vi "Initialize.vi"(6 "Reset (True)":bool=TRUE, 7 "Serial Configuration":T1={"Baud Rate"=9600, "Parity"=0, "Data Bits"=7, "Stop Bits"=10, "Flow Control"=0} {"Flow Control" items=["None", "XON/XOFF", "RTS/CTS", "XON/XOFF & RTS/CTS", "DTR/DSR", "XON/XOFF & DTR/DSR"]; "Stop Bits" items=["1.0"=10, "1.5"=15, "2.0"=20]; "Data Bits" items=["7"=7, "8"=8]; "Parity" items=["None", "Odd", "Even", "Mark", "Space"]; "Baud Rate" items=["300"=300, "600"=600, "1200"=1200, "2400"=2400, "4800"=4800, "9600"=9600, "19200"=19200]}, 8 "error in (no error)":errorcluster, 9 "Error Query (False)":bool, 10 "ID Query (True)":bool=TRUE, 11 "VISA resource name":refnum<visa-resource-name>) -> (0 "error out":errorcluster, 3 "VISA resource name out":refnum<visa-resource-name>)   [LabVIEW 2018, in "Keithley 2600 Series.lvlib"]
doc: "Establishes communication with the instrument and optionally performs an instrument identification query and/or an instrument reset. It also places the instrument in a default state needed for other instrument driver operations. Therefore, call this VI before calling other instrument driver VIs for this instrument. Generally, you need to call the Initialize VI only once at the beginning of an application."
uses:
  Keithley 2600 Series.lvlib
  GlobalVariables.vi
panel:
  # "(c) 2008 Keithley Instruments, Inc.  ALL RIGHTS RESERVED."
  # "Automatic"
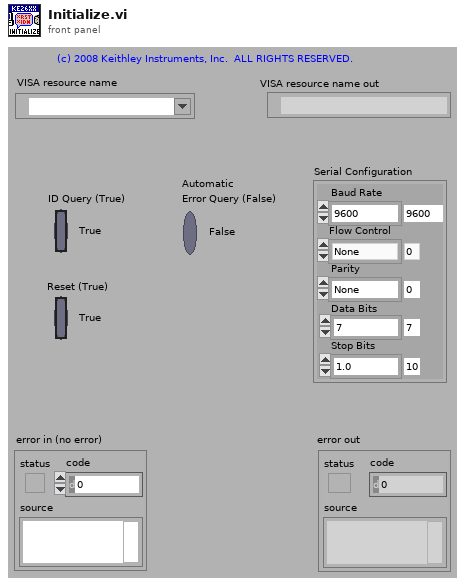
[diagram p1: front panel]
types:
  T1 = cluster{"Baud Rate":u32, "Parity":u16, "Data Bits":u16, "Stop Bits":u16, "Flow Control":u16}
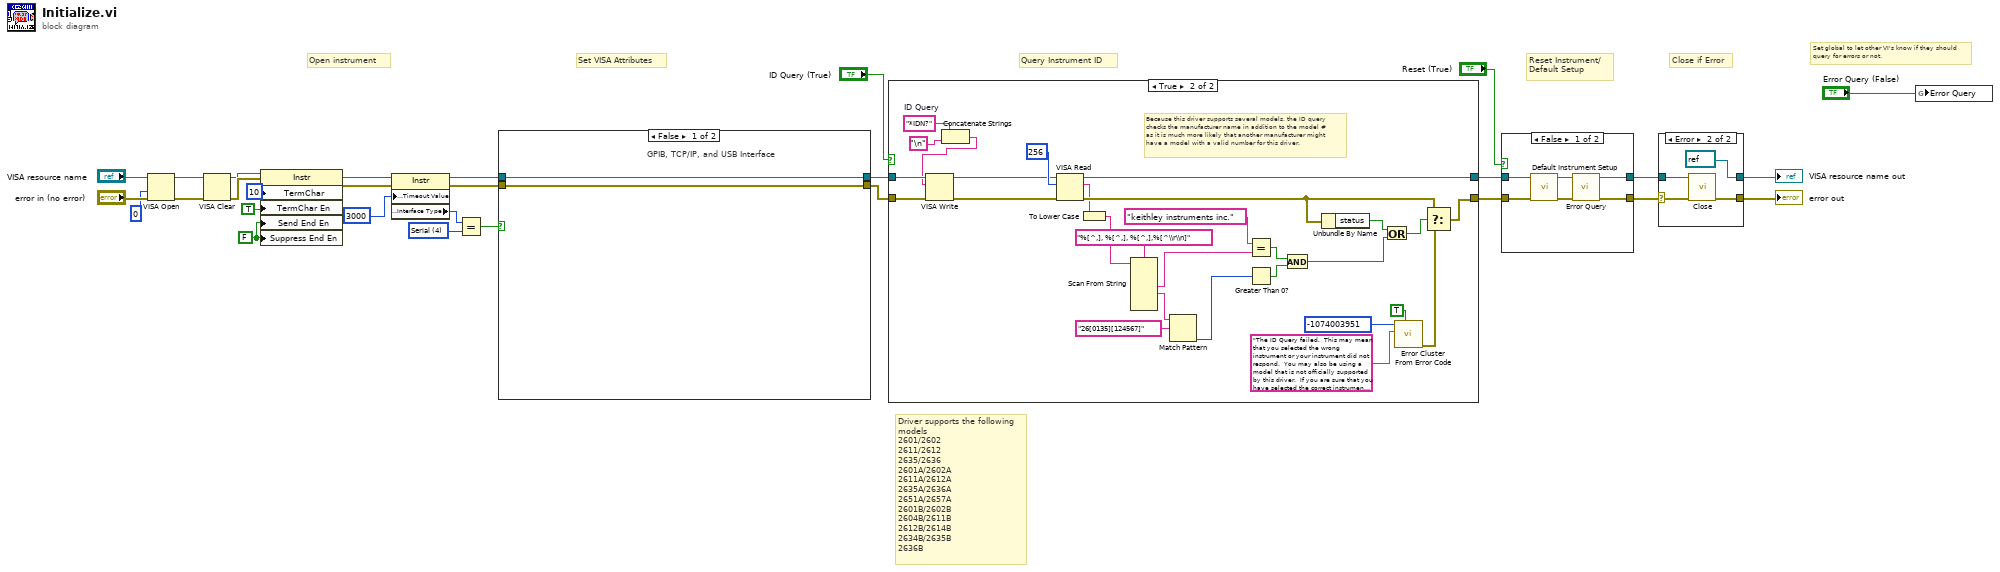
[diagram p0: block diagram]
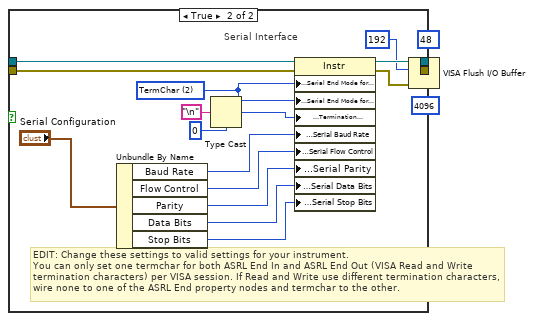
[diagram p2: hidden frame]
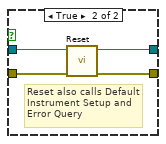
[diagram p4: hidden frame]
diagram:
  w1 = FALSE ("Message Based Settings:Suppress End Enable")
  w16 = u16 4 items=["GPIB"=1, "VXI"=2, "GPIB-VXI"=3, "Serial"=4, "PXI"=5, "TCPIP"=6, "USB"=7] ("Interface Information:Interface Type")
  # "Driver supports the following models\n2601/2602\n2611/2612\n2635/2636\n2601A/2602A\n2611A/2612A\n2635A/2636A\n2651A/2657A\n2601B/2602B\n2604B/2611B\n2612B/2614B\n2634B/2635B\n2636B"
  # "Set global to let other VI's know if they should\nquery for errors or not."
  # "Set VISA Attributes"
  # "Close if Error"
  # "Query Instrument ID"
  # "Reset Instrument/\nDefault Setup"
  # "Open instrument"
  n1 = VISA Open(access mode=u32 0, error in (no error)="error in (no error)", VISA resource name="VISA resource name") -> (VISA resource name=w14:refnum<visa-resource-name>, error out=w13:errorcluster)  [unwired: 2 out]
  n2 = VISA Clear(VISA resource name=w14, error in (no error)=w13) -> (VISA resource name out=w4:refnum<visa-resource-name>, error out=w5:errorcluster)
  n3 = property class="Instr"(reference=w4, error in=w5, "TermChar"=u8 10 ("Message Based Settings:Termination Character"), "TermChar En"=TRUE ("Message Based Settings:Termination Character Enable"), "Send End En"=w1, "Suppress End En"=w1) -> (reference out=w3:refnum<visa-resource-name>, error out=w2:errorcluster)
  n4 = property class="Instr"(reference=w3, error in=w2, "General Settings:Timeout Value"=u32 3000) -> (reference out=w19:refnum<visa-resource-name>, error out=w18:errorcluster, "Interface Information:Interface Type"=w23:u16)
  n5 = Equal?(x=w23, y=w16) -> (x = y?=w17:bool)
  n6 = case shown="False" w17 {
    tunnel: [w30 w49] -> w21
    tunnel: [w31 w46] -> w20
    tunnel: w19 -> [w30 w51]
    tunnel: w18 -> [w31 w52]
    frame False {
      # "GPIB, TCP/IP, and USB Interface"
    }
    frame True {
      w39 = u16 2 items=["None", "LastBit", "TermChar"] ("Serial Settings:Serial End Mode for Reads")
      # "EDIT: Change these settings to valid settings for your instrument.\nYou can only set one termchar for both ASRL End In and ASRL End Out (VISA Read and Write termination characters) per VISA session. If Read and Write use different termination characters, wire none to one of the ASRL End property nodes and termchar to the other."
      # "Serial Interface"
      n7 = Unbundle By Name("Serial Configuration") -> ("Baud Rate"=w37:u32, "Flow Control"=w33:u16, "Parity"=w35:u16, "Data Bits"=w36:u16, "Stop Bits"=w32:u16)
      n8 = Type Cast(type=u8 0, x="\n" ("Line Feed Constant")) -> (*(type *) &x=w38:u8)
      n9 = property class="Instr"(reference=w51, error in=w52, "Serial Settings:Serial End Mode for Reads"=w39, "Serial Settings:Serial End Mode for Writes"=w39, "Message Based Settings:Termination Character"=w38, "Serial Settings:Serial Baud Rate"=w37, "Serial Settings:Serial Flow Control"=w33, "Serial Settings:Serial Parity"=w35, "Serial Settings:Serial Data Bits"=w36, "Serial Settings:Serial Stop Bits"=w32) -> (reference out=w45:refnum<visa-resource-name>, error out=w48:errorcluster)
      n10 = VISA Flush I/O Buffer(VISA resource name=w45, mask (16)=u16 192, error in (no error)=w48) -> (VISA resource name out=w50:refnum<visa-resource-name>, error out=w47:errorcluster)
      n11 = VISA Set I/O Buffer Size(VISA resource name=w50, mask (16)=u16 48, size (4096)=u32 4096 ("size (0)"), error in (no error)=w47) -> (VISA resource name out=w49:refnum<visa-resource-name>, error out=w46:errorcluster)
    }
  }
  n12 = case shown="True" "ID Query (True)" {
    tunnel: [w53 w82] -> w28
    tunnel: [w54 w79] -> w29
    tunnel: w21 -> [w54 w80]
    tunnel: w20 -> [w53 w81]
    frame False {
    }
    frame True {
      w63 = "*IDN?"  # ID Query
      # "Because this driver supports several models, the ID query\nchecks the manufacturer name in addition to the model #\nas it is much more likely that another manufacturer might\nhave a model with a valid number for this driver."
      n13 = Concatenate Strings(w63, "\n") -> (w61:string)
      n14 = VISA Write(VISA resource name=w80, write buffer=w61, error in (no error)=w81) -> (VISA resource name out=w56:refnum<visa-resource-name>, error out=w55:errorcluster)  [unwired: 1 out]
      n15 = VISA Read(VISA resource name=w56, byte count=u32 256, error in (no error)=w55) -> (VISA resource name out=w79:refnum<visa-resource-name>, read buffer=w74:string, error out=w77:errorcluster)  [unwired: 1 out]
      n16 = To Lower Case(string=w74) -> (all lower case string=w68:string)
      n17 = Scan From String(format string="%[^,], %[^,], %[^,],%[^\\r\\n]", input string=w68) -> (output 1=w66:string, output 2=w64:string)  [unwired: 4 in, 7 out]
      n18 = Match Pattern(string=w64, regular expression="26[0135][124567]") -> (offset past match=w72:i32)  [unwired: 4 out]
      n19 = Equal?(x="keithley instruments inc." ("regular expression"), y=w66) -> (x = y?=w65:bool)
      n20 = Greater Than 0?(x=w72) -> (x > 0?=w71:bool)
      n21 = And(x=w65, y=w71) -> (x .and. y?=w70:bool)
      n22 = Unbundle By Name(w77) -> ("status"=w76:bool)
      n23 = Or(x=w76, y=w70) -> (x .or. y?=w75:bool)
      n24 = call "Error Cluster From Error Code.vi"("show call chain? (False)"=TRUE, "error message (\"\")"="The ID Query failed.  This may mean that you selected the wrong instrument or your instrument did not respond.  You may also be using a model that is not officially supported by this driver.  If you are sure that you have selected the correct instrument and it is responding, try disabling the ID Query." ("Source (VI Name)"), "error code (0)"=-1074003951 ("Code")) -> ("error out"=w78:errorcluster)  [unwired: 1 in, 5 out]
      n25 = Select(t=w77, s=w75, f=w78) -> (s? t:f=w82:errorcluster)
    }
  }
  n26 = case shown="False" "Reset (True)" {
    tunnel: w28 -> [w87 w89]
    tunnel: [w84 w92] -> w9
    tunnel: w29 -> [w88 w90]
    tunnel: [w85 w91] -> w10
    frame False {
      n27 = call "Default Instrument Setup.vi"("error in (no error)"=w87, "VISA resource name"=w88) -> ("error out"=w83:errorcluster, "VISA resource name out"=w86:refnum<visa-resource-name>)  [unwired: 8 out]
      n28 = call "Error Query.vi"("error in (no error)"=w83, "VISA resource name"=w86) -> ("error out"=w84:errorcluster, "VISA resource name out"=w85:refnum<visa-resource-name>)  [unwired: 8 out]
    }
    frame True {
      # "Reset also calls Default Instrument Setup and Error Query"
      n29 = call "Reset.vi"("error in (no error)"=w89, "VISA resource name"=w90) -> ("error out"=w92:errorcluster, "VISA resource name out"=w91:refnum<visa-resource-name>)  [unwired: 8 out]
    }
  }
  n30 = case shown="Error" w9 {
    selector: w9 -> [w93 w96]
    tunnel: w10 -> [w94 w97]
    tunnel: [w94 refnum<visa-resource-name> refnum ("VISA resource name out")] -> w12
    tunnel: [w93 w98] -> w11
    frame No Error {
    }
    frame Error {
      n31 = call "Close.vi"("error in (no error)"=w96, "VISA resource name"=w97) -> ("error out"=w98:errorcluster)  [unwired: 9 out]
    }
  }
  "VISA resource name out" <- w12
  "error out" <- w11
  n32 = global write "GlobalVariables.vi" "Error Query"("Error Query (False)") -> ()
